vi "pruebaDaq.vi"() -> ()   [LabVIEW 2011]
panel:
  in  "Boolean":bool
  in  "breake 2":bool
  in  "Aumentar":bool
  in  "stop":bool
  out "alarma de temperatura":bool
  out "Temperatura":i32(knob) scale=0.0..5.0
  out "Encendido":bool
  out "Cuarta":bool
  out "Tercera":bool
  out "Segunda":bool
  out "Primera":bool
  out "Acelerador":bool
  out "Breake":bool
  out "Velocidad":i32(knob) scale=1.0..220.0
  # "Se tiene que generar la temperatura del auto de acuerdoa la\nvelocidad:\n1-70  temp 1-2\n70-130 temp 1-4\n130-  temp 1-5\nesto es una entrada que se escribe en la temperatura \n y salida analógica que se ingresa del valor de la temperatura\na la DAQ.\n\nEl acelerador cada vez que se pulsa el boton que sera \nuna entrada de la daq aumenta la velocidad en 10.\nSi se presiona el boton del breake se rebaja la velocidad en 5.\n\ndebera de producirse 4 salidas digitales para \nrepreentar cada uno de los cambios usando led\n1-30 primera\n31-50 segunda\n50-80 tercera\n80- cuarta.\n\nla alarma de la temperatura se enciende solo si esta \nsube arriba de 3 enciende un led en la daq , la que es una\nsalida digital."
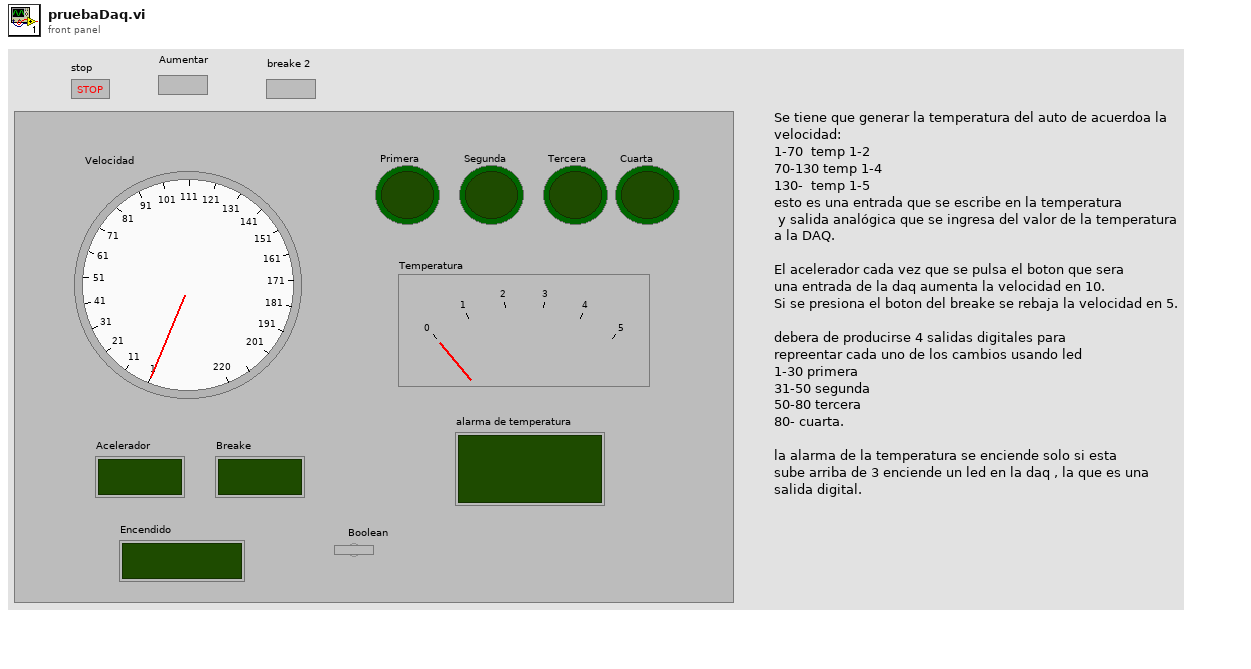
[diagram p1: front panel]
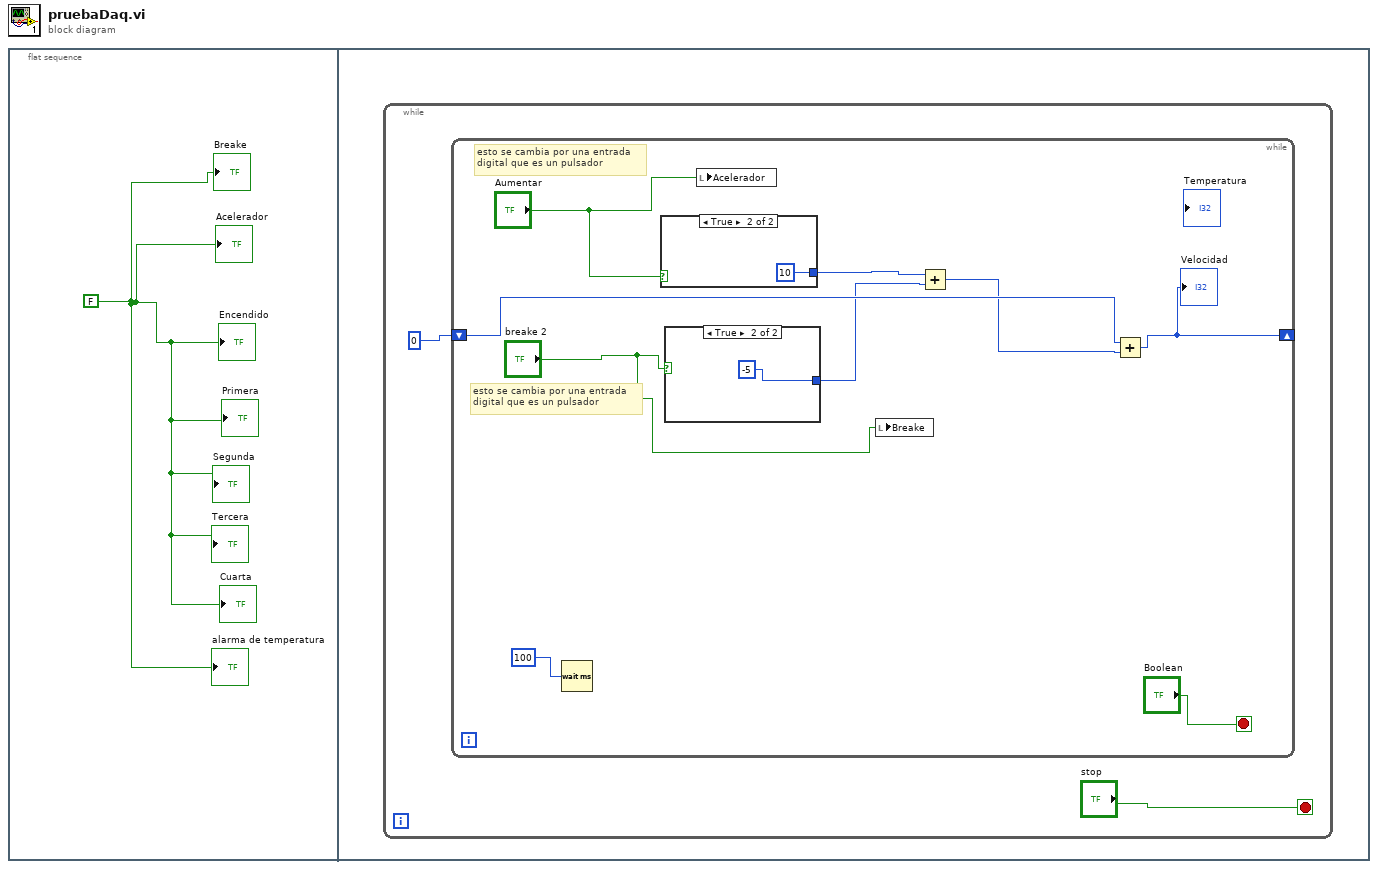
[diagram p0: block diagram]
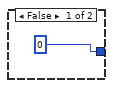
[diagram p2: hidden frame]
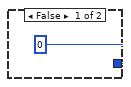
[diagram p3: hidden frame]
diagram:
  n1 = flat-sequence {
    frame #0 {
      w1 = FALSE
      "Breake" <- w1
      "Acelerador" <- w1
      "Encendido" <- w1
      "Primera" <- w1
      "Segunda" <- w1
      "Tercera" <- w1
      "Cuarta" <- w1
      "alarma de temperatura" <- w1
    }
    frame #1 {
      n2 = while {
        stop <- "stop" stop-if-true
        n3 = while {
          shift-right: [w8] -> _
          shift-left: 0 -> [w9]
          stop <- "Boolean" stop-if-true
          # "esto se cambia por una entrada \ndigital que es un pulsador"
          # "esto se cambia por una entrada \ndigital que es un pulsador"
          n4 = Wait (ms)(milliseconds to wait=100) -> ()  [unwired: 1 out]
          n5 = case shown="True" "Aumentar" {
            tunnel: [0 10] -> w10
            frame False {
            }
            frame True {
            }
          }
          n6 = case shown="True" "breake 2" {
            tunnel: [0 -5] -> w7
            frame False {
            }
            frame True {
            }
          }
          n7 = local write "Acelerador"("Aumentar") -> ()
          n8 = local write "Breake"("breake 2") -> ()
          n9 = Add(x=w10, y=w7) -> (x+y=w6:i32)
          n10 = Add(x=w9, y=w6) -> (x+y=w8:i32)
          "Velocidad" <- w8
        }
      }
    }
  }
